vi "stimulate_and_record.vi"(3 "SSH password":string, 4 "Transfer and Run Date Folder After Experiment":bool, 5 "SSH user name":string, 6 "Tags":string, 7 "Frames":i32, 8 "Convert Power to Voltage":bool, 9 "voltages/power":dbl[](array[numeric]), 10 "parameters":string[](array[string]), 11 "parameters headers":string[](array[string])) -> ()   [LabVIEW 2014]
uses:
  <vilib>/vision/driver/NI_Vision_Acquisition_Software.lvlib
  <vilib>/userdefined/High Color/IMAQdx.ctl
  <vilib>/Utility/file.llb/Write To Spreadsheet File (DBL).vi
  <vilib>/Utility/file.llb/Read Delimited Spreadsheet (string).vi
  <vilib>/Utility/file.llb/Write To Spreadsheet File (string).vi
panel:
  out "Error":string
  out "Save Directory":path
  out "Buffer Number Out":u32
  out "Image":T1(plugin-control)
  in  "stop":bool
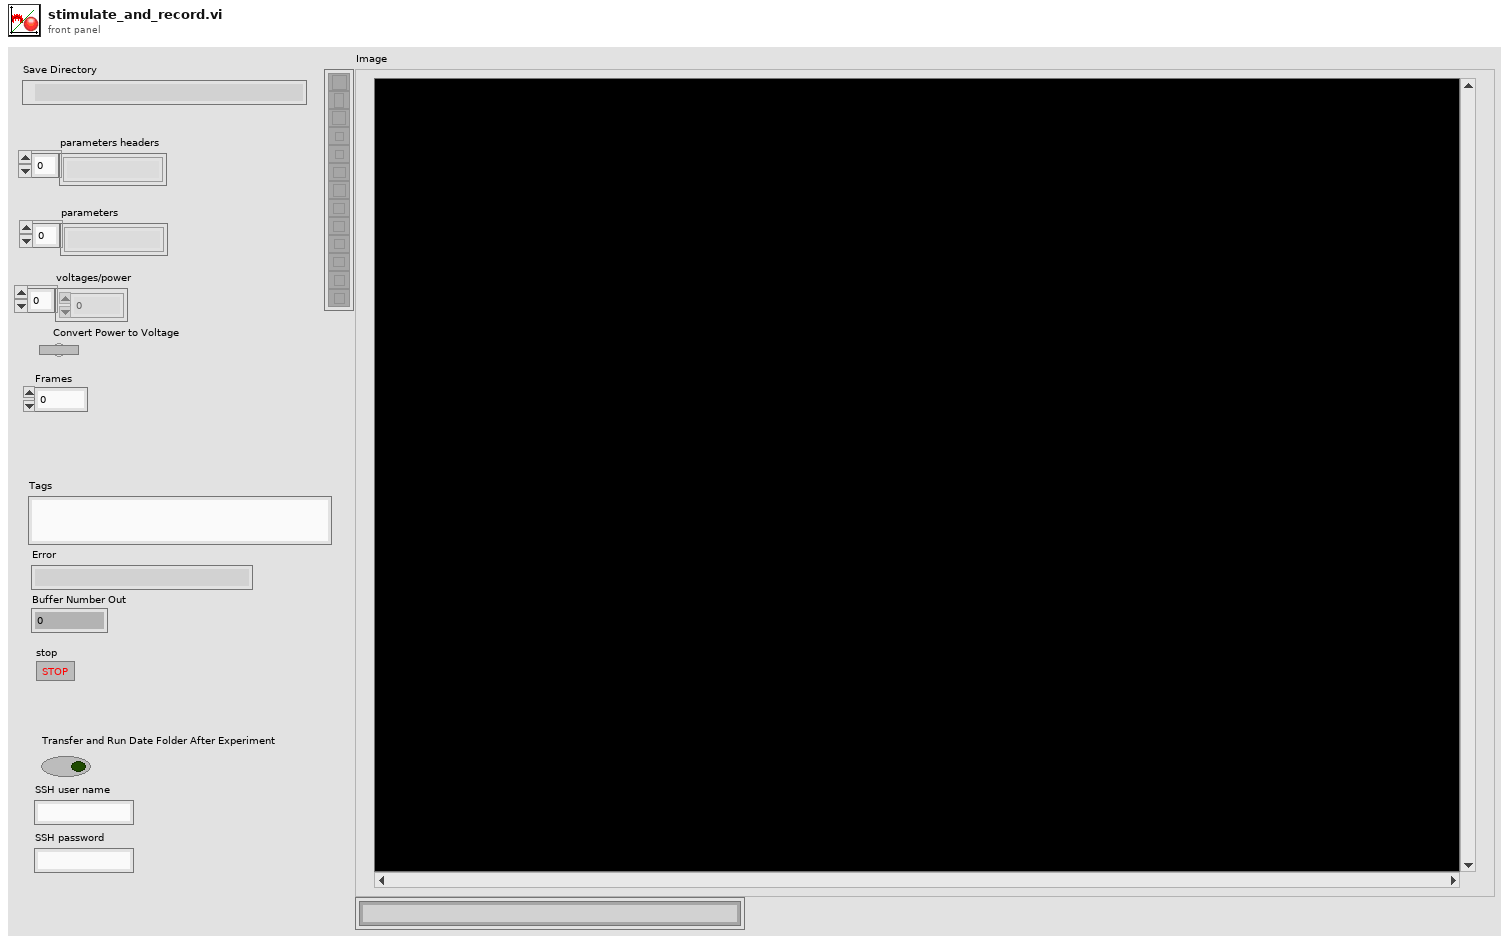
[diagram p1: front panel]
types:
  T1 = typedef "IMAQ Image.ctl" = refnum<image>
  T2 = typedef "IMAQdx.ctl" = refnum<k21>
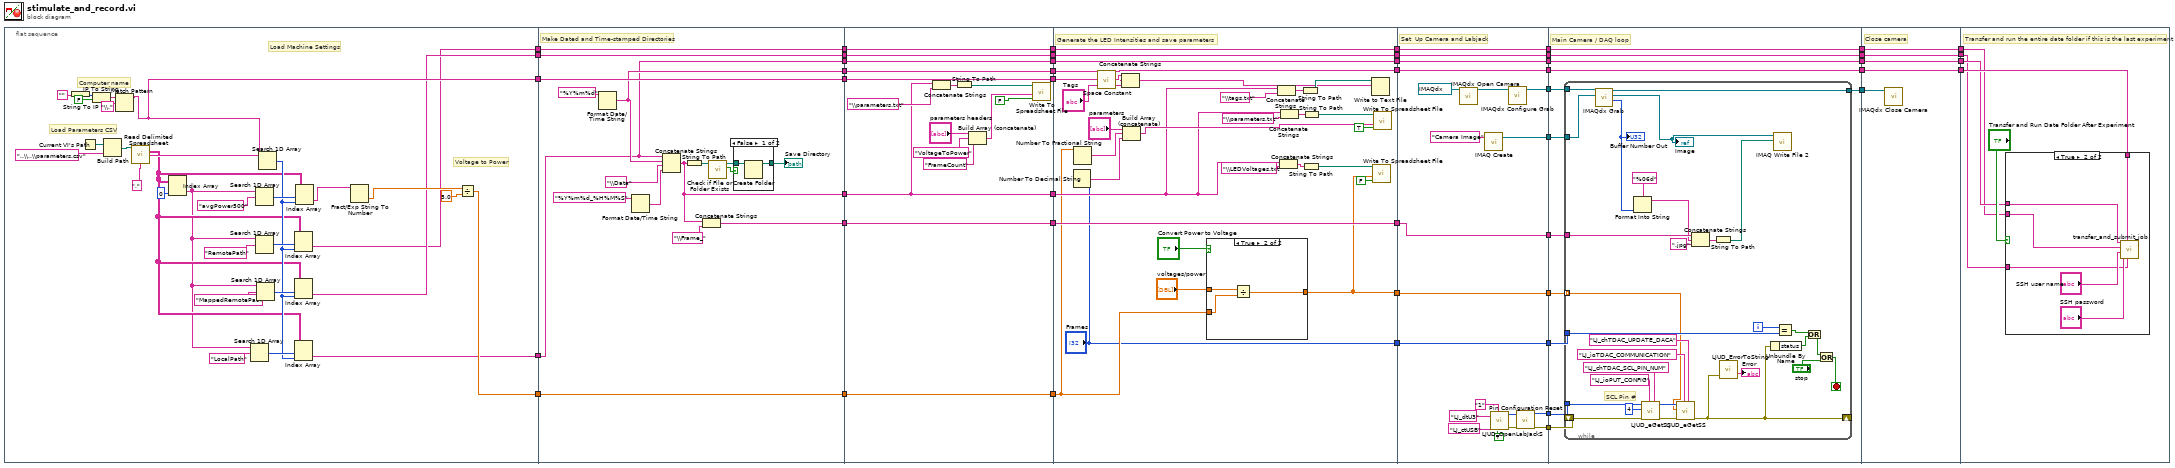
[diagram p0: block diagram]
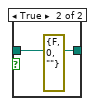
[diagram p2: hidden frame]
diagram:
  n1 = flat-sequence {
    tunnel: [w70] -> w37
    tunnel: [w67] -> w36
    tunnel: [w52] -> w27
    tunnel: [w51] -> w26
    tunnel: [w50] -> w25
    tunnel: [w95] -> w16
    tunnel: [w94] -> w14
    tunnel: [w93] -> w12
    tunnel: [w92] -> w10
    tunnel: [w91] -> w8
    tunnel: [w90] -> w6
    tunnel: [w89] -> w4
    tunnel: [w88] -> w2
    tunnel: w25 -> [w89]
    tunnel: w26 -> [w88]
    tunnel: w27 -> [w90]
    tunnel: w36 -> [w92]
    tunnel: w37 -> [w93]
    tunnel: w16 -> [w114]
    tunnel: [w114] -> w15
    tunnel: w14 -> [w99]
    tunnel: [w99] -> w13
    tunnel: w12 -> [w113]
    tunnel: [w113] -> w11
    tunnel: w10 -> [w112]
    tunnel: [w112] -> w9
    tunnel: w8 -> [w111]
    tunnel: [w111] -> w7
    tunnel: w6 -> [w110]
    tunnel: [w110] -> w5
    tunnel: w4 -> [w109]
    tunnel: [w109] -> w3
    tunnel: w2 -> [w108]
    tunnel: [w108] -> w1
    tunnel: w15 -> [w142]
    tunnel: [w142] -> w42
    tunnel: [w120] -> w40
    tunnel: ["Frames"] -> w39
    tunnel: w13 -> [w134]
    tunnel: w11 -> [w116]
    tunnel: w9 -> [w130]
    tunnel: w7 -> [w126]
    tunnel: [w126] -> w32
    tunnel: [w125] -> w28
    tunnel: w5 -> [w125]
    tunnel: [w124] -> w21
    tunnel: w3 -> [w124]
    tunnel: [w123] -> w17
    tunnel: w1 -> [w123]
    tunnel: w42 -> [w163]
    tunnel: [w165] -> w48
    tunnel: [w164] -> w47
    tunnel: [w163] -> w46
    tunnel: [w155] -> w44
    tunnel: [w154] -> w43
    tunnel: [w159] -> w41
    tunnel: w40 -> [w159]
    tunnel: w39 -> [w158]
    tunnel: [w158] -> w38
    tunnel: [w152] -> w33
    tunnel: w32 -> [w152]
    tunnel: [w151] -> w29
    tunnel: w28 -> [w151]
    tunnel: [w150] -> w22
    tunnel: w21 -> [w150]
    tunnel: [w149] -> w18
    tunnel: w17 -> [w149]
    tunnel: w48 -> [w180]
    tunnel: w47 -> [w179]
    tunnel: w46 -> [w178]
    tunnel: [w177] -> w45
    tunnel: w44 -> [w176]
    tunnel: w43 -> [w175]
    tunnel: w41 -> [w174]
    tunnel: w38 -> [w173]
    tunnel: [w172] -> w34
    tunnel: w33 -> [w172]
    tunnel: [w171] -> w30
    tunnel: w29 -> [w171]
    tunnel: [w170] -> w23
    tunnel: w22 -> [w170]
    tunnel: [w169] -> w19
    tunnel: w18 -> [w169]
    tunnel: w45 -> [w215]
    tunnel: [w214] -> w35
    tunnel: w34 -> [w214]
    tunnel: [w213] -> w31
    tunnel: w30 -> [w213]
    tunnel: [w212] -> w24
    tunnel: w23 -> [w212]
    tunnel: [w211] -> w20
    tunnel: w19 -> [w211]
    tunnel: w35 -> [w219]
    tunnel: w31 -> [w218]
    tunnel: w24 -> [w216]
    tunnel: w20 -> [w217]
    frame #0 {
      # "Voltage to Power"
      # "Load Parameters CSV"
      # "Computer name"
      # "Load Machine Settings"
      n2 = String To IP(1:"") -> (0:w78:u32)
      n3 = Current VI's Path() -> (path=w73:path)
      n4 = IP To String(1:FALSE, 2:w78) -> (0:w75:string)
      n5 = Build Path(base path=w73, name or relative path="..\\..\\parameters.csv") -> (appended path=w69:path)
      n6 = Match Pattern(string=w75, regular expression="\\.") -> (before substring=w67:string)  [unwired: 1 in, 3 out]
      n7 = call-poly <vilib>:"Read Delimited Spreadsheet.vi"("file path (dialog if empty)"=w69, "delimiter (\\t)"=",") -> ("all rows"=w53:string[][], "first row"=w66:string[])  [unwired: 8 in, 4 out]
      n8 = Index Array(array=w53, index (col)=0) -> (element=w49:string[])  [unwired: 1 in]
      n9 = Search 1D Array(1D array=w49, element="LocalPath") -> (index of element=w55:i32)  [unwired: 1 in]
      n10 = Search 1D Array(1D array=w49, element="RemotePath") -> (index of element=w60:i32)  [unwired: 1 in]
      n11 = Search 1D Array(1D array=w49, element="avgPower500") -> (index of element=w61:i32)  [unwired: 1 in]
      n12 = Search 1D Array(1D array=w49, element="MappedRemotePath") -> (index of element=w59:i32)  [unwired: 1 in]
      n13 = Search 1D Array(1D array=w66, element=w67) -> (index of element=w54:i32)  [unwired: 1 in]
      n14 = Index Array(array=w53, index (row)=w60, index (col)=w54) -> (element=w50:string)
      n15 = Index Array(array=w53, index (row)=w59, index (col)=w54) -> (element=w51:string)
      n16 = Index Array(array=w53, index (row)=w55, index (col)=w54) -> (element=w52:string)
      n17 = Index Array(array=w53, index (row)=w61, index (col)=w54) -> (element=w58:string)
      n18 = Fract/Exp String To Number(string=w58) -> (number=w57:dbl)  [unwired: 3 in, 1 out]
      n19 = Divide(x=w57, y=5.0) -> (x/y=w70:dbl)
    }
    frame #1 {
      # "Make Dated and Time-stamped Directories"
      n20 = Format Date/Time String(time format string (%c)="%Y%m%d") -> (date/time string=w91:string)  [unwired: 2 in]
      n21 = Format Date/Time String(time format string (%c)="%Y%m%d_%H%M%S") -> (date/time string=w82:string)  [unwired: 2 in]
      n22 = Concatenate Strings(w90, w91, "\\Data", w82) -> (w94:string)
      n23 = String To Path(string=w94) -> (path=w81:path)
      n24 = Concatenate Strings(w94, "\\Frame_") -> (w95:string)
      n25 = call <vilib>:"Check if File or Folder Exists.vi"("path"=w81) -> ("file or folder exists?"=w86:bool, "dup path"=w85:path)  [unwired: 8 in, 1 out]
      n26 = case shown="False" w86 {
        tunnel: [w96 w98] -> w80
        tunnel: w85 -> [w97 w98]
        frame False {
          n27 = Create Folder(path (use dialog)=w97) -> (created path=w96:path)  [unwired: 2 in, 2 out]
        }
        frame True {
          (unwired) errorcluster {"status"=FALSE, "code"=0, "source"=""} ("error out")
        }
      }
      "Save Directory" <- w80
    }
    frame #2 {
      n28 = Concatenate Strings(w99, "\\parameters.txt") -> (w107:string)
      n29 = String To Path(string=w107) -> (path=w106:path)
      n30 = Build Array (concatenate)("parameters headers", "VoltageToPower", "FrameCount") -> (w103:string[])
      n31 = call-poly <vilib>:"Write To Spreadsheet File.vi"("append to file? (new file:F)"=FALSE, "1D data"=w103, "file path (dialog if empty)"=w106) -> ()  [unwired: 5 in, 1 out]
    }
    frame #3 {
      # "Generate the LED Intensities and save parameters"
      n32 = Number To Decimal String(number="Frames") -> (decimal integer string=w118:string)  [unwired: 1 in]
      n33 = Number To Fractional String(number=w116) -> (F-format string=w117:string)  [unwired: 3 in]
      n34 = call <vilib>:"Space Constant.vi"() -> ("String"=w128:string)
      n35 = Concatenate Strings(w130, w128, "Tags") -> (w127:string)
      n36 = Build Array (concatenate)("parameters", w117, w118) -> (w135:string[])
      n37 = case shown="True" "Convert Power to Voltage" {
        tunnel: "voltages/power" -> [w145 w148]
        tunnel: [w145 w146] -> w120
        tunnel: w116 -> [_ w147]
        frame False {
        }
        frame True {
          n38 = Divide(x=w148, y=w147) -> (x/y=w146:dbl[])
        }
      }
      n39 = Concatenate Strings(w134, "\\tags.txt") -> (w132:string)
      n40 = Concatenate Strings(w134, "\\LEDVoltages.txt") -> (w144:string)
      n41 = Concatenate Strings(w134, "\\parameters.txt") -> (w139:string)
      n42 = String To Path(string=w132) -> (path=w131:path)
      n43 = String To Path(string=w144) -> (path=w143:path)
      n44 = String To Path(string=w139) -> (path=w138:path)
      n45 = Write to Text File(file (use dialog)=w131, text=w127) -> ()  [unwired: 2 in, 3 out]
      n46 = call-poly <vilib>:"Write To Spreadsheet File.vi"("append to file? (new file:F)"=FALSE, "1D data"=w120, "file path (dialog if empty)"=w143) -> ()  [unwired: 5 in, 1 out]
      n47 = call-poly <vilib>:"Write To Spreadsheet File.vi"("append to file? (new file:F)"=TRUE, "1D data"=w135, "file path (dialog if empty)"=w138) -> ()  [unwired: 5 in, 1 out]
    }
    frame #4 {
      # "Set  Up Camera and Labjack"
      n48 = call <vilib>:"IMAQdx Open Camera.vi"("Session In"=T2 "cam0") -> ("Session Out"=w167:T2)  [unwired: 9 in, 1 out]
      n49 = call "IMAQ Create"("Image Name"="Camera Image") -> ("New Image"=w164:T1)  [unwired: 4 in, 1 out]
      n50 = call "LJUD_OpenLabJackS.vi"("FirstFound"=TRUE, "Address"="1" ("DeviceType"), "ConnectionType"="LJ_ctUSB", "DeviceType"="LJ_dtU3") -> ("error out"=w153:errorcluster, "Handle"=w156:i32)  [unwired: 5 in, 1 out]
      n51 = call <vilib>:"IMAQdx Configure Grab.vi"("Session In"=w167) -> ("Session Out"=w165:T2)  [unwired: 9 in, 1 out]
      n52 = call "Pin Configuration Reset.vi"("error in"=w153, "Handle In"=w156) -> ("error out"=w154:errorcluster, "Handle Out"=w155:i32)  [unwired: 8 in]
    }
    frame #5 {
      # "Main Camera / DAQ loop"
      n53 = while {
        tunnel: w180 -> [w210]
        tunnel: [w209] -> w177
        tunnel: w179 -> [w208]
        tunnel: w178 -> [w206]
        tunnel: w176 -> [w183]
        shift-right: [w184] -> _
        shift-left: w175 -> [w182]
        tunnel: w174 -> [w181] mode=indexing
        tunnel: w173 -> [w192]
        i -> [w193]
        stop <- w199 stop-if-true
        # "SCL Pin #"
        n54 = call <vilib>:"IMAQdx Grab.vi"("Image In"=w208, "Session In"=w210) -> ("Buffer Number Out"=w202:u32, "Image Out"=w207:T1, "Session Out"=w209:T2)  [unwired: 6 in, 1 out]
        "Image" <- w207
        "Buffer Number Out" <- w202
        n55 = Format Into String(format string="%06d" ("string"), w202) -> (resulting string=w201:string)  [unwired: 2 in, 1 out]
        n56 = call "LJUD_eGetSS.vi"("Channel"="LJ_chTDAC_SCL_PIN_NUM", "IOType"="LJ_ioPUT_CONFIG", "error in"=w182, "Value Write"=4, "Handle In"=w183) -> ("error out"=w185:errorcluster, "Handle Out"=w188:i32)  [unwired: 4 in, 1 out]
        n57 = call "LJUD_eGetSS.vi"("Channel"="LJ_chTDAC_UPDATE_DACA", "IOType"="LJ_ioTDAC_COMMUNICATION", "error in"=w185, "Value Write"=w181, "Handle In"=w188) -> ("error out"=w184:errorcluster)  [unwired: 4 in, 2 out]
        n58 = Concatenate Strings(w206, w201, ".jpg" ("string")) -> (w204:string)
        n59 = String To Path(string=w204) -> (path=w203:path)
        n60 = call "LJUD_ErrorToString.vi"("error in"=w184) -> ("String"=→"Error":string)  [unwired: 10 in]
        n61 = Unbundle By Name(w184) -> ("status"=w196:bool)
        n62 = call-poly "IMAQ Write File 2"("File Path"=w203, "Image"=w207) -> ()  [unwired: 8 in, 2 out]
        n63 = Equal?(x=w193, y=w192) -> (x = y?=w195:bool)
        n64 = Or(x=w195, y=w196) -> (x .or. y?=w194:bool)
        n65 = Or(x=w194, y="stop") -> (x .or. y?=w199:bool)
      }
    }
    frame #6 {
      # "Close camera"
      n66 = call <vilib>:"IMAQdx Close Camera.vi"("Session In"=w215) -> ()  [unwired: 10 in, 1 out]
    }
    frame #7 {
      # "Transfer and run the entire date folder if this is the last experiment"
      n67 = case shown="True" "Transfer and Run Date Folder After Experiment" {
        tunnel: w219 -> [_ w224]
        tunnel: w218 -> [_ w223]
        tunnel: w217 -> [_ w222]
        tunnel: w216 -> [_ w221]
        frame False {
        }
        frame True {
          n68 = call "transfer_and_submit_job.vi"("Mapped Remote Directory Path"=w222, "Date Folder"=w224, "Password"="SSH password", "Username"="SSH user name", "Remote Data Directory"=w221, "Local Data Directory"=w223) -> ()  [unwired: 6 in]
        }
      }
    }
  }
